vi "Open.vi"(8 "error in (no error)":errorcluster, 11 "TcpServer In":refnum<class "TcpServer.lvclass">) -> (0 "error out":errorcluster, 3 "TcpServer Out":refnum<class "TcpServer.lvclass">)   [LabVIEW 2022 SP3, in "TcpSocket.lvlib" / "TcpServer.lvclass"]
uses:
  TcpServer.lvclass
  C:/Users/jakub/repos/gh/sw4sys/lv-tcp-socket/TcpSocket/Source/TcpSocket/TcpSocket/TcpSocket.lvclass
  TcpSocket/TcpSocket.lvclass/TcpSocket.ctl
  TcpSocket/Read Address.vi
  TcpSocket/Read Port.vi
  TcpSocket/Read OpenTimeout.vi
  TcpSocket/Write Connection.vi
  TcpSocket/Write Port.vi
  TcpServer.lvclass/TcpServer.ctl
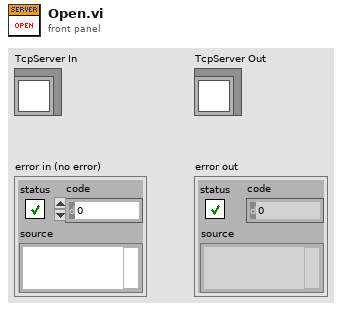
[diagram p1: front panel]
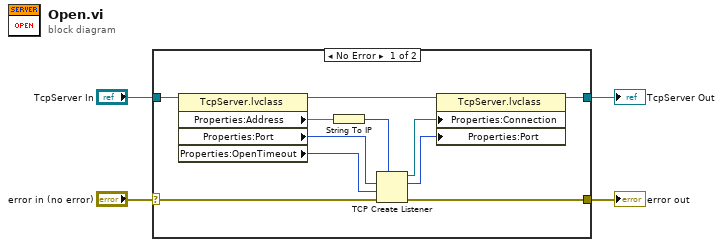
[diagram p0: block diagram]
diagram:
  n1 = case shown="No Error" "error in (no error)" {
    selector: "error in (no error)" -> [w15 w17]
    tunnel: [w13 w17] -> w3
    tunnel: "TcpServer In" -> [w12 w16]
    tunnel: [w7 w16] -> w1
    frame No Error {
      n2 = property class="TcpServer.lvclass"(reference=w12) -> (reference out=w8:refnum<class "TcpServer.lvclass">, "Properties:Address"=w11:string, "Properties:Port"=w10:u16, "Properties:OpenTimeout"=w9:i32)  [unwired: 1 in, 1 out]
      n3 = String To IP(1:w11) -> (0:w14:u32)
      n4 = TCP Create Listener(7:w14, 8:w15, 9:w9, 10:w10) -> (0:w13:errorcluster, 2:w5:u16, 3:w6:refnum<k5>)  [unwired: 1 in]
      n5 = property class="TcpServer.lvclass"(reference=w8, "Properties:Connection"=w6, "Properties:Port"=w5) -> (reference out=w7:refnum<class "TcpServer.lvclass">)  [unwired: 1 in, 1 out]
    }
    frame Error {
    }
  }
  "error out" <- w3
  "TcpServer Out" <- w1
